vi "Read T.vi"(8 "error in (no error)":errorcluster, 11 "ePAS Cell Data in":refnum<class "ePAS Cell Data.lvclass">) -> (0 "error out":errorcluster, 2 "T":dbl[](array[numeric]), 3 "ePAS Cell Data out":refnum<class "ePAS Cell Data.lvclass">)   [LabVIEW 2014, in "ePAS Library.lvlib" / "ePAS Cell Data.lvclass"]
uses:
  ePAS Cell Data.lvclass
  ePAS Cell Data.lvclass/ePAS Cell Data.ctl
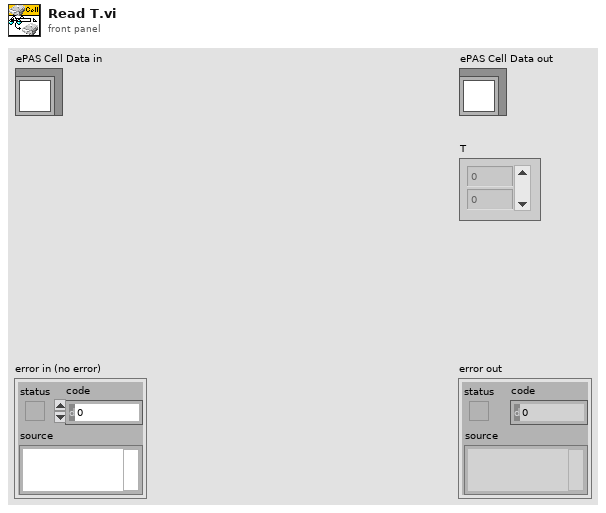
[diagram p1: front panel]
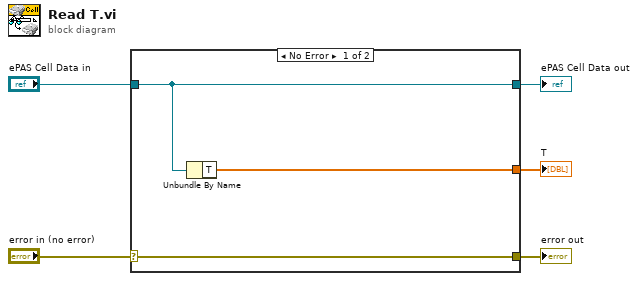
[diagram p0: block diagram]
diagram:
  n1 = case shown="No Error" "error in (no error)" {
    selector: "error in (no error)" -> [w8 w9]
    tunnel: [w8 w9] -> w4
    tunnel: [w7 w10] -> w2
    tunnel: "ePAS Cell Data in" -> [w7 w10]
    tunnel: [w6 _] -> w1
    frame No Error {
      n2 = Unbundle By Name(w7) -> ("T"=w6:dbl[])
    }
    frame Error {
    }
  }
  "error out" <- w4
  "ePAS Cell Data out" <- w2
  "T" <- w1
